vi "Acquisition Message Loop.vi"(8 "error in (no error)":errorcluster, 11 "Message Queues":T1) -> (0 "error out":errorcluster)   [LabVIEW 2018, in "Acquisition.lvlib"]
doc: "Message loop for handling messages pertaining to the acquisition of data from the hardware."
uses:
  Acquisition.lvlib
  support/Message Queue/All Message Queues.ctl
  support/Message Queue/Message Cluster.ctl
  controls/Acquired Data.ctl
  Hardware Configuration.ctl
  support/Message Queue/Message Queue.lvlib
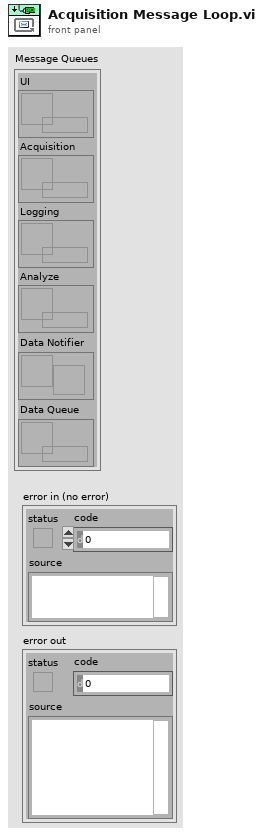
[diagram p1: front panel]
types:
  T1 = typedef "Message Queue.lvlib/All Message Queues.ctl" = cluster{"UI":refnum<queue>, "Acquisition":refnum<queue>, "Logging":refnum<queue>, "Analyze":refnum<queue>, "Data Notifier":refnum<notifier>, "Data Queue":refnum<queue>}
  T2 = typedef "Acquisition.lvlib/Hardware Configuration.ctl" = cluster{"DAQmx AI Channels":tag, "Aquatrak COM Port":refnum<visa-resource-name>, "Ring Time Task":refnum<k21>}
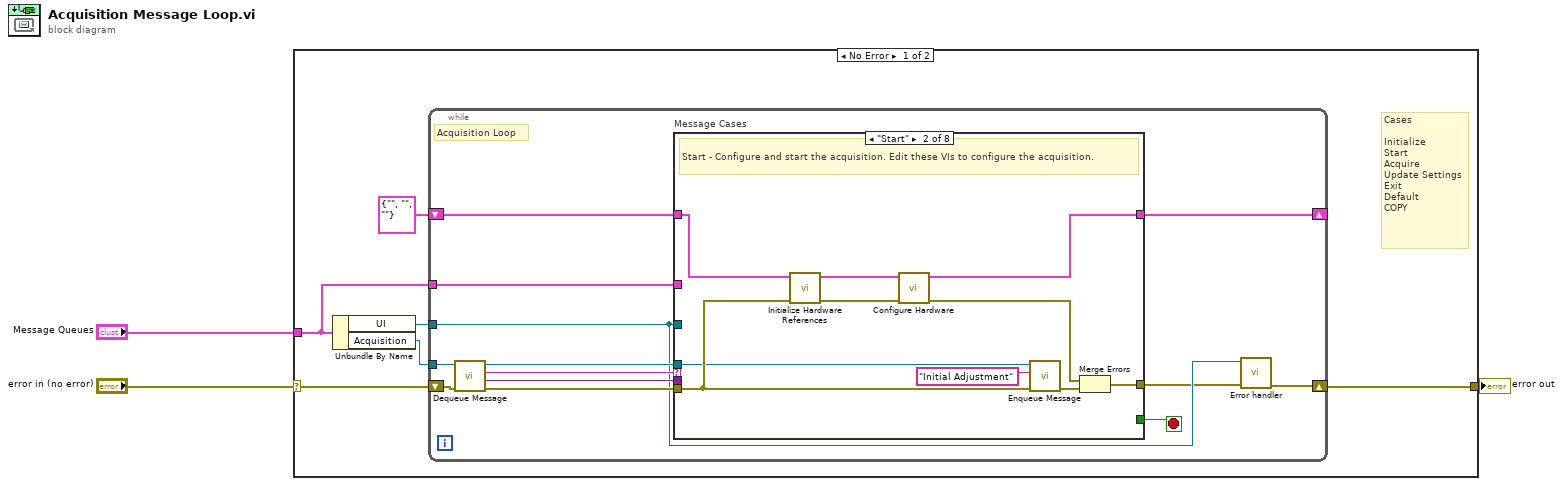
[diagram p0: block diagram]
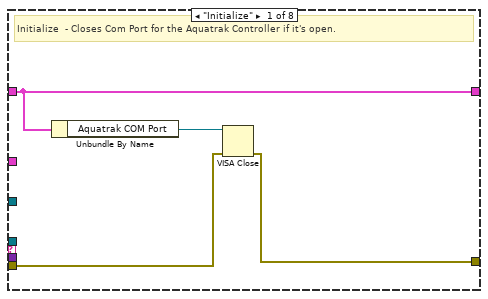
[diagram p2: hidden frame]
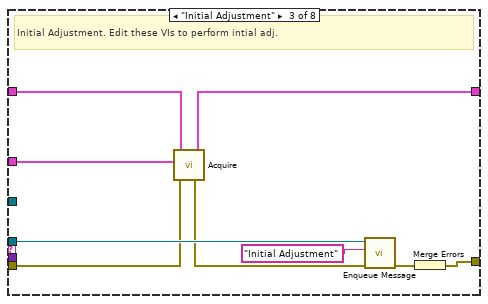
[diagram p3: hidden frame]
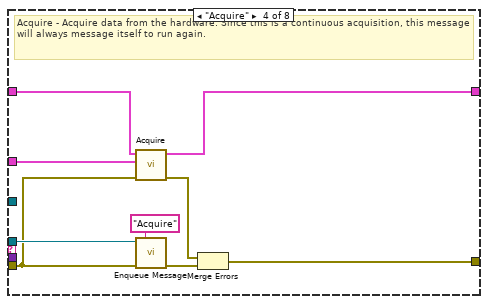
[diagram p4: hidden frame]
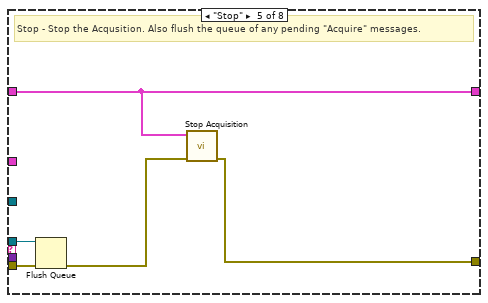
[diagram p5: hidden frame]
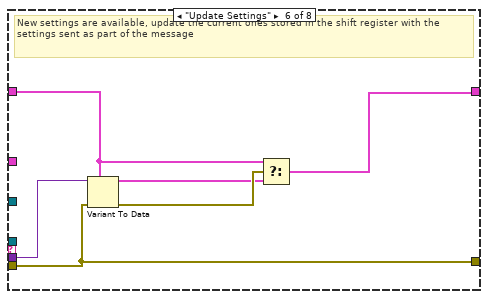
[diagram p6: hidden frame]
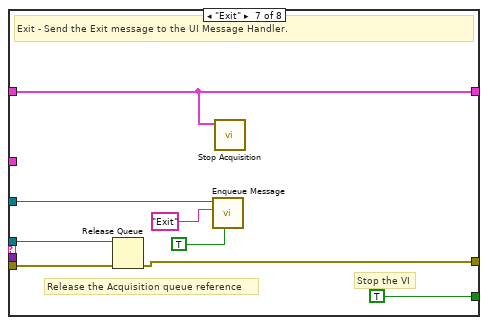
[diagram p7: hidden frame]
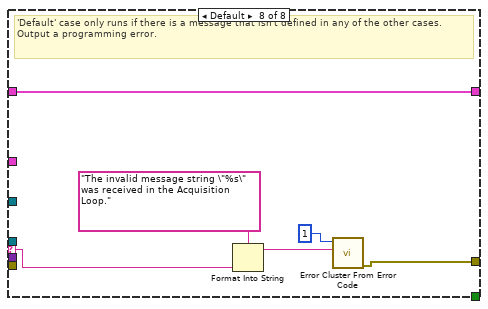
[diagram p8: hidden frame]
diagram:
  n1 = case shown="No Error" "error in (no error)" {
    selector: "error in (no error)" -> [w7 w80]
    tunnel: "Message Queues" -> [w5 _]
    tunnel: [w4 w80] -> w3
    frame No Error {
      # "Cases\n\nInitialize\nStart\nAcquire\nUpdate Settings\nExit\nDefault\nCOPY"
      n2 = Unbundle By Name(w5) -> ("UI"=w6:refnum<queue>, "Acquisition"=w9:refnum<queue>)
      n3 = while {
        tunnel: w9 -> [w14]
        shift-right: [w21] -> _
        shift-left: T2 {"DAQmx AI Channels"="", "Aquatrak COM Port"="", "Ring Time Task"=""} ("Data Cluster") -> [w22]
        shift-right: [w10] -> w4
        shift-left: w7 -> [w19]
        tunnel: w6 -> [w13]
        tunnel: w5 -> [w12]
        stop <- w20 stop-if-true
        # "Acquisition Loop"
        n4 = call "Dequeue Message.vi"("error in (no error)"=w19, "Message Queue"=w14) -> ("error out"=w18:errorcluster, "Message Data"=w16:variant, "Message"=w17:string, "dup Message Queue"=w15:refnum<queue>)  [unwired: 6 in]
        n5 = case "Message Cases" shown="\"Start\"" w17 {
          selector: w17 -> [_ _ _ _ _ _ _ w77]
          tunnel: w15 -> [_ w33 w43 w53 w55 _ w67 _]
          tunnel: w18 -> [w23 w35 w38 w52 w59 w60 w71 _]
          tunnel: [w24 w36 w45 w47 w58 w60 w68 w75] -> w11
          tunnel: w22 -> [w26 w27 w41 w48 w57 w62 w66 w79]
          tunnel: [w26 w29 w39 w50 w57 w61 w66 w79] -> w21
          tunnel: [_ _ _ _ _ _ TRUE _] -> w20
          tunnel: w16 -> [_ _ _ _ _ w65 _ _]
          tunnel: w13 -> [_ _ _ _ _ _ w72 _]
          tunnel: w12 -> [_ _ w40 w46 _ _ _ _]
          frame "Initialize" {
            # "Initialize  - Closes Com Port for the Aquatrak Controller if it's open."
            n6 = Unbundle By Name(w26) -> ("Aquatrak COM Port"=w25:refnum<visa-resource-name>)
            n7 = VISA Close(VISA resource name=w25, error in (no error)=w23) -> (error out=w24:errorcluster)
          }
          frame "Start" {
            # "Start - Configure and start the acquisition. Edit these VIs to configure the acquisition."
            n8 = call "Initialize Hardware References.vi"("error in (no error)"=w35, "Hardware Resources in"=w27) -> ("error out"=w32:errorcluster, "Hardware Resources out"=w30:T2)  [unwired: 8 in]
            n9 = call "Configure Hardware.vi"("error in (no error)"=w32, "Hardware Resources in"=w30) -> ("error out"=w31:errorcluster, "Hardware Resources out"=w29:T2)  [unwired: 8 in]
            n10 = call "Enqueue Message.vi"("error in (no error)"=w35, "Message"="Initial Adjustment", "Message Queue"=w33) -> ("error out"=w34:errorcluster)  [unwired: 7 in, 1 out]
            n11 = Merge Errors(w31, w34) -> (w36:errorcluster)
          }
          frame "Initial Adjustment" {
            # "Initial Adjustment. Edit these VIs to perform intial adj."
            n12 = call "Acquire.vi"("error in (no error)"=w38, "Message Queues"=w40, "Hardware Resources in"=w41) -> ("error out"=w37:errorcluster, "Hardware Resources out"=w39:T2)  [unwired: 7 in]
            n13 = call "Enqueue Message.vi"("error in (no error)"=w37, "Message"="Initial Adjustment", "Message Queue"=w43) -> ("error out"=w44:errorcluster)  [unwired: 7 in, 1 out]
            n14 = Merge Errors(w44) -> (w45:errorcluster)
          }
          frame "Acquire" {
            # "Acquire - Acquire data from the hardware. Since this is a continuous acquisition, this message will always message itself to run again."
            n15 = call "Acquire.vi"("error in (no error)"=w52, "Message Queues"=w46, "Hardware Resources in"=w48) -> ("error out"=w51:errorcluster, "Hardware Resources out"=w50:T2)  [unwired: 7 in]
            n16 = call "Enqueue Message.vi"("error in (no error)"=w52, "Message"="Acquire", "Message Queue"=w53) -> ("error out"=w54:errorcluster)  [unwired: 7 in, 1 out]
            n17 = Merge Errors(w51, w54) -> (w47:errorcluster)
          }
          frame "Stop" {
            # "Stop - Stop the Acqusition. Also flush the queue of any pending \"Acquire\" messages."
            n18 = Flush Queue(queue=w55, error in (no error)=w59) -> (error out=w56:errorcluster)  [unwired: 2 out]
            n19 = call "Stop Acquisition.vi"("error in (no error)"=w56, "Hardware Resources in"=w57) -> ("error out"=w58:errorcluster)  [unwired: 9 in]
          }
          frame "Update Settings" {
            # "New settings are available, update the current ones stored in the shift register with the settings sent as part of the message"
            n20 = Variant To Data(error in=w60, type=w62, Variant=w65) -> (data=w63:T2, error out=w64:errorcluster)
            n21 = Select(t=w62, s=w64, f=w63) -> (s? t:f=w61:T2)
          }
          frame "Exit" {
            # "Release the Acquisition queue reference"
            # "Stop the VI"
            # "Exit - Send the Exit message to the UI Message Handler."
            n22 = Release Queue(queue=w67, error in (no error)=w71) -> (error out=w68:errorcluster)  [unwired: 1 in, 2 out]
            n23 = call "Enqueue Message.vi"("Priority Message? (F)"=TRUE, "Message"="Exit", "Message Queue"=w72) -> ()  [unwired: 7 in, 2 out]
            n24 = call "Stop Acquisition.vi"("Hardware Resources in"=w66) -> ()  [unwired: 10 in, 1 out]
          }
          frame Default {
            # "'Default' case only runs if there is a message that isn't defined in any of the other cases.  Output a programming error."
            n25 = Format Into String(format string="The invalid message string \"%s\" was received in the Acquisition Loop." ("Invalid Acquisition Message"), w77) -> (resulting string=w74:string)  [unwired: 2 in, 1 out]
            n26 = call <vilib>:"Error Cluster From Error Code.vi"("error message (\"\")"=w74, "error code (0)"=1) -> ("error out"=w75:errorcluster)  [unwired: 7 in]
          }
        }
        n27 = call "Error handler.vi"("error in (no error)"=w11, "Queue in"=w13) -> ("error out"=w10:errorcluster)  [unwired: 9 in]
      }
    }
    frame Error {
      # "Handle Acquisition Errors right here...buddy."
    }
  }
  "error out" <- w3
